vi "Main.vi"(8 "error in":errorcluster, 11 "UI Cam Basler in":refnum<class "UI Cam Basler.lvclass">) -> (0 "error out":errorcluster, 3 "UI Cam Basler out":refnum<class "UI Cam Basler.lvclass">)   [LabVIEW 2023, in "UI Cam Basler.lvclass"]
doc: "The Queued Message Handler of a Worker."
uses:
  UI Cam Basler.lvclass
  <vilib>/userDefined/High Color/IMAQdx.ctl
  C:/Program Files (x86)/National Instruments/LabVIEW 2023/vi.lib/addons/_Workers/Library/Classes/Worker/Worker.lvclass
  Data Image.ctl
  <vilib>/vision/Image Controls.llb/IMAQ Image.ctl
  UI Cam Basler.lvclass/UI Cam Basler.ctl
  <vilib>/addons/_Workers/Library/Classes/Worker/Worker.lvclass/Worker.ctl
  Initialization Data.ctl
  <vilib>/MGI/Panel Manager - .NET Panels/MDI/MDI Container/MDI Container.lvclass
  <vilib>/MGI/Panel Manager/Panel/Window Position/Reference Position/Alignment.ctl
  <vilib>/MGI/Panel Manager/Panel/Window Position/Reference Position/Horizontal Alignment.ctl
  <vilib>/MGI/Panel Manager/Panel/Window Position/Reference Position/Vertical Alignment.ctl
  <vilib>/MGI/Panel Manager/Panel/Window Position/Reference Position/Size/Reference Size/Reference Size.lvclass/Reference Size.ctl
  <vilib>/Utility/miscctls.llb/LVMinMaxIncTypeDef.ctl
  <vilib>/MGI/Panel Manager/Panel/Window Position/Reference Position/Size/Reference Size/Reference Size.vi
  <vilib>/MGI/Panel Manager/Panel/Window Position/Reference Position/Size/Reference Size/Reference Size.lvclass
  C:/Program Files (x86)/National Instruments/LabVIEW 2023/vi.lib/MGI/Panel Manager/Panel/Window Position/Reference Position/Size/Size.lvclass
  <vilib>/MGI/Panel Manager - .NET Panels/MDI/MDI Panel/MDI Panel.lvclass
  C:/Program Files (x86)/National Instruments/LabVIEW 2023/vi.lib/MGI/Panel Manager/Panel/Panel/Panel.lvclass
  Acq Cam Basler/Acq Cam Basler.lvclass
  <vilib>/MGI/Panel Manager - .NET Panels/MDI/MDI Panel/MDI Panel_Sized Window.vi
  <userlib>/LV-TOML/lib/Write TOML File (TOML).vi
  <vilib>/addons/_Workers/Library/Classes/Message/Enqueue Message to Queue.vi
  <vilib>/addons/_Workers/Library/Classes/Message/Enqueue Message to Self v2.vi
  <vilib>/addons/_Workers/Library/Classes/Worker/Worker.lvclass
  <vilib>/MGI/Panel Manager/Panel/Window Position/Reference Position/Reference Position.lvclass
  <vilib>/MGI/Panel Manager/Panel/Panel.lvlib
  <vilib>/MGI/Panel Manager/Panel/Panel/Panel.lvclass
  <userlib>/LV-TOML/lib/LV-TOML.lvlib
  <vilib>/addons/_Workers/Library/Classes/Message/Message.lvclass
  C:/Program Files (x86)/National Instruments/LabVIEW 2023/vi.lib/addons/_Workers/Library/Classes/Workers Object/Workers Object.lvclass
  C:/Users/flepetit/Desktop/CamView-mdi-LV/Workers/Acq Cam Basler/Acq Cam Basler.lvclass
  C:/Users/flepetit/Desktop/CamView-mdi-LV/Workers/UI Cam Basler/UI Cam Basler.lvclass
  C:/Program Files (x86)/National Instruments/LabVIEW 2023/vi.lib/MGI/Panel Manager/Panel/Panel/Window/Window.lvclass
  C:/Program Files (x86)/National Instruments/LabVIEW 2023/vi.lib/MGI/Panel Manager - .NET Panels/MDI/MDI Panel/MDI Panel.lvclass
  C:/Program Files (x86)/National Instruments/LabVIEW 2023/vi.lib/MGI/Panel Manager/Panel/Window Position/Reference Position/Size/Reference Size/Reference Size.lvclass
panel:
  out "Image":T1(plugin-control)
  in  "Commande onglets":T2(tab)
  in  "Save Config":bool
  in  "Start":bool
  in  "Stop":bool
  in  "Camera Name":T3
  out "FPS":dbl
  in  "Gain":dbl=100.0 min=100.0 max=1023.0 step=1.0
  in  "Shutter(us)":dbl=4.0 min=4.0 max=1000000.0 step=1.0
  in  "ROI":bool
  in  "toolbar?":bool
  in  "Palette":u32(ring)=5 items=["Grayscale", "Binary", "Gradient", "Rainbow", "Temperature", "User Defined", "Binary 16 Bit", "Gradient 16 Bit", "Rainbow 16 Bit", "Temperature 16 Bit", "User Defined 16 Bit"]
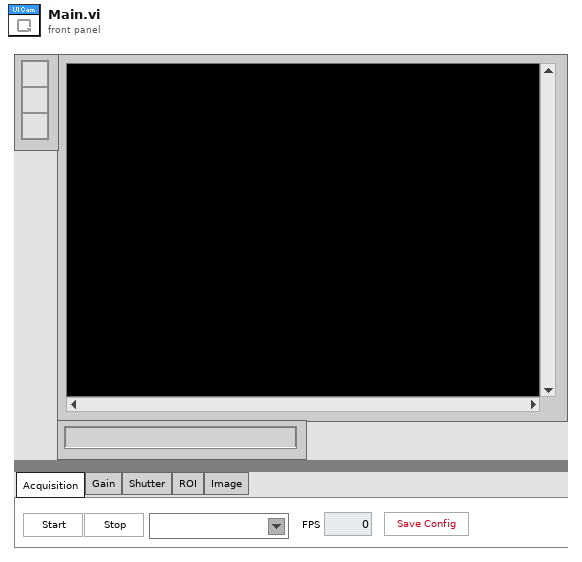
[diagram p1: front panel]
types:
  T1 = typedef "IMAQ Image.ctl" = refnum<image>
  T2 = enum32{"Acquisition", "Gain", "Shutter", "ROI", "Image"}
  T3 = typedef "IMAQdx.ctl" = refnum<k21>
  T4 = typedef "UI Cam Basler.lvclass/Data Image.ctl" = cluster{"Image Out":T1, "FPS":dbl}
  T5 = typedef "UI Cam Basler.lvclass/Initialization Data.ctl" = cluster{"Module Name":string, "Container":refnum<class "MDI Container.lvclass">, "Offset":cluster{"Horizontal":i16, "Vertical":i16}, "Width Scale":dbl, "Height Scale":dbl, "Alignment":T6}
  T6 = typedef "Panel.lvlib/Reference Position.lvclass/Alignment.ctl" = cluster{"Horizontal":T7, "Vertical":T8}
  T7 = typedef "Panel.lvlib/Reference Position.lvclass/Horizontal Alignment.ctl" = enum16{"Left", "Center", "Right"}
  T8 = typedef "Panel.lvlib/Reference Position.lvclass/Vertical Alignment.ctl" = enum16{"Top", "Center", "Bottom"}
  T9 = typedef "LVMinMaxIncTypeDef.ctl" = cluster{"Minimum":dbl, "Maximum":dbl, "Increment":dbl}
  T10 = typedef "UI Cam Basler.lvclass/Parsed Data Acquisition.ctl" = cluster{"Config Acquisition":cluster{"Camera name":string, "Gain":dbl, "Shutter(us)":dbl, "ROI":bool, "ROI coor":T11, "Palette":u32, "ModelName":string}}
  T11 = typedef "IMAQ Rectangle" = cluster{"Left":i32, "Top":i32, "Right":i32, "Bottom":i32, "Rotation":dbl}
  T12 = typedef "LV-TOML.lvlib/TOML Value.ctl" = cluster{"type":enum16{"Table", "Array", "String", "Integer", "Float", "Boolean", "Offset Date-Time", "Local Date-Time", "Local Date", "Local Time", "Path"}, "value":variant}
  T13 = typedef "Workers.lvlib/Case Label.ctl" = string
  T14 = typedef "ROI Descriptor" = cluster{"Global Rectangle":i32[], "Contours":cluster{"ID":enum32{"External", "Internal"}, "Type":u32, "Coordinates":i32[]}[]}
  T15 = cluster{"Global Rectangle":i32[], "Contours":cluster{"Contour Type":u32, "ROI Type":u32, "Points":i32[]}[]}
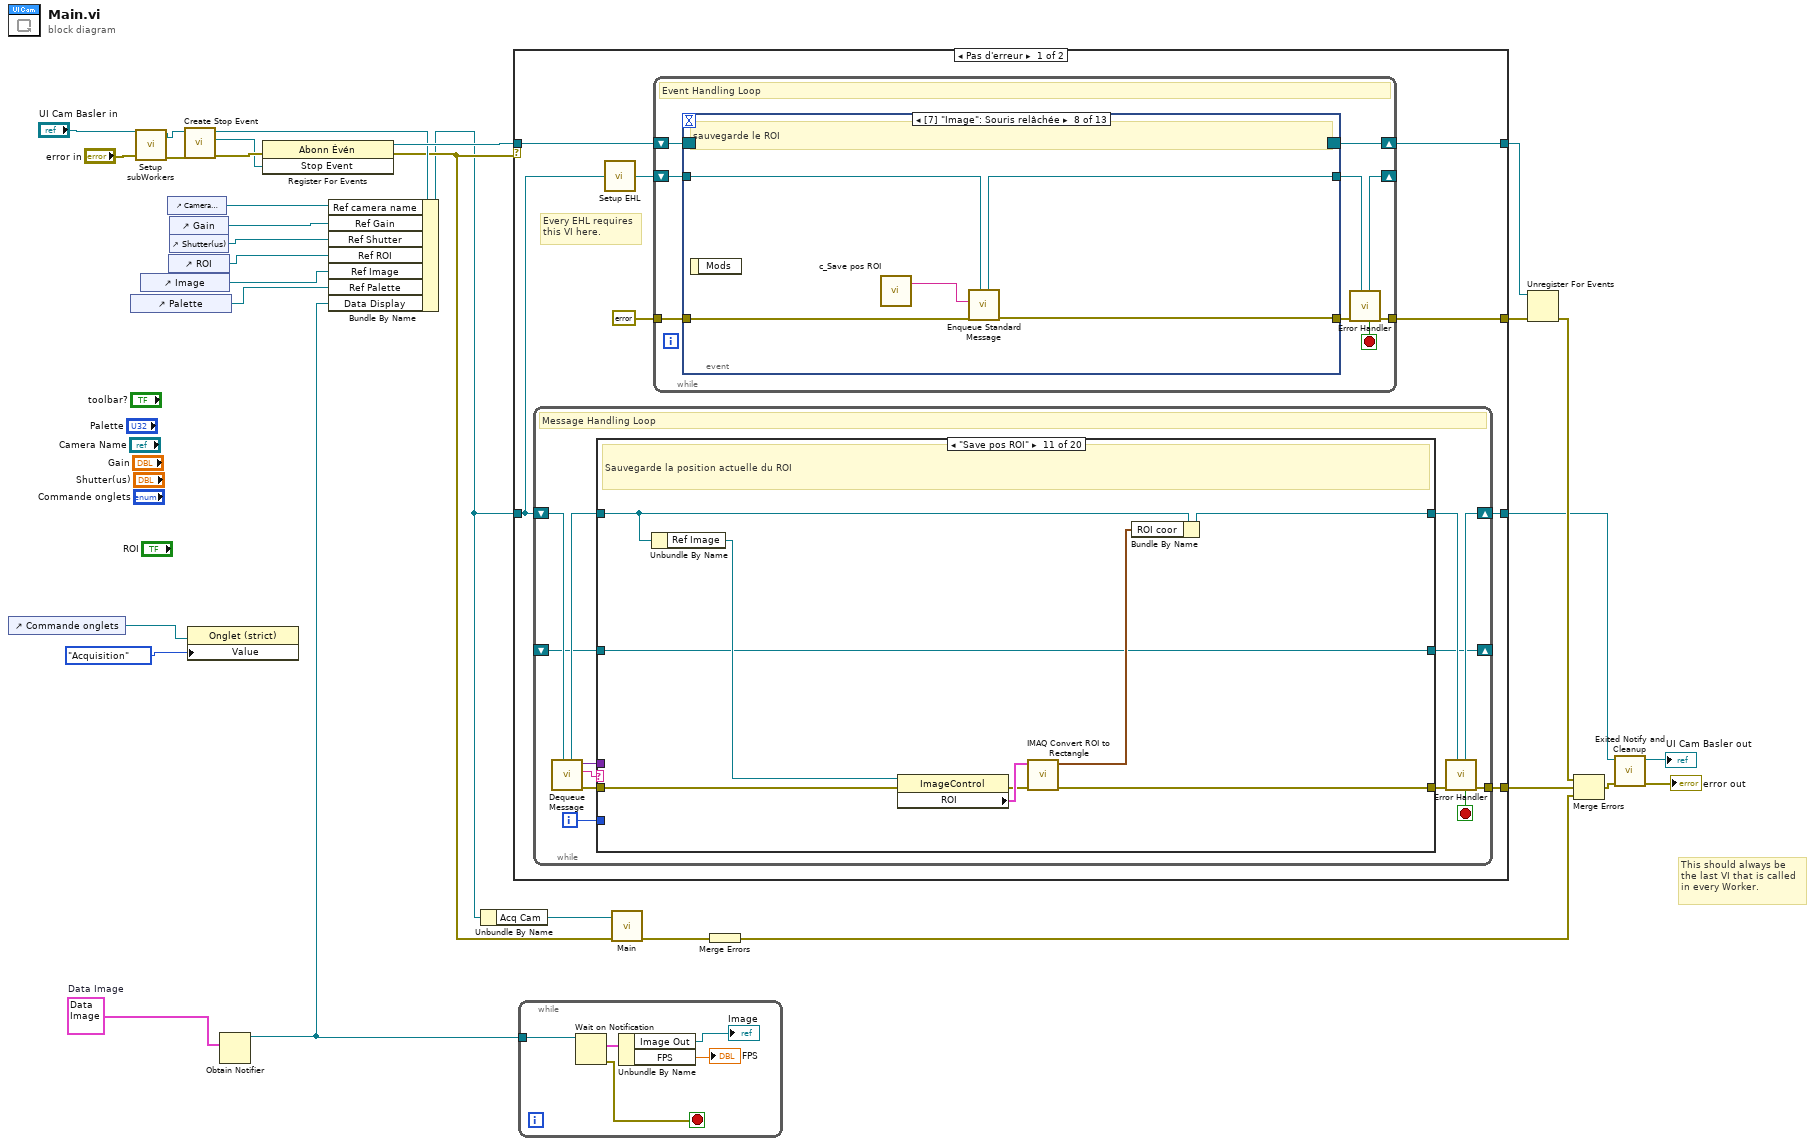
[diagram p0: block diagram]
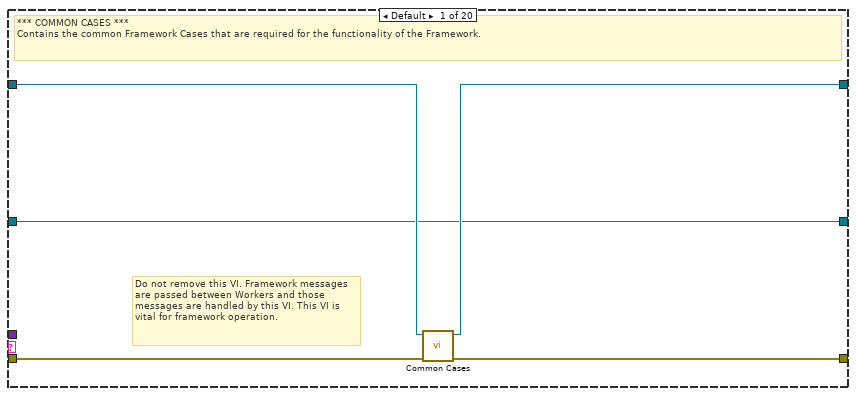
[diagram p2: hidden frame]
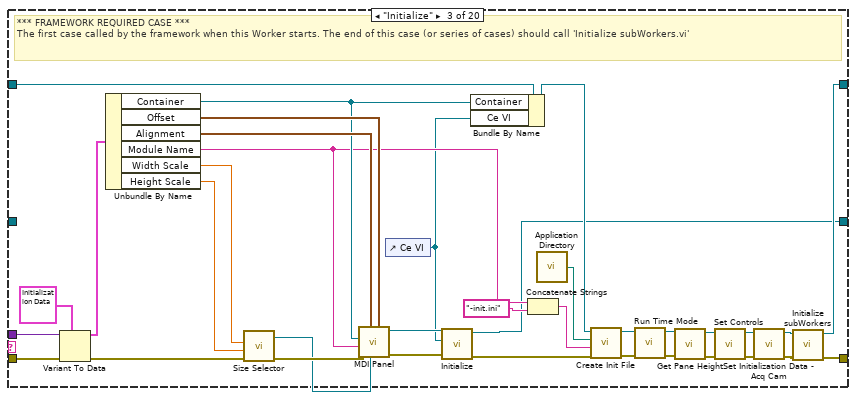
[diagram p4: hidden frame]
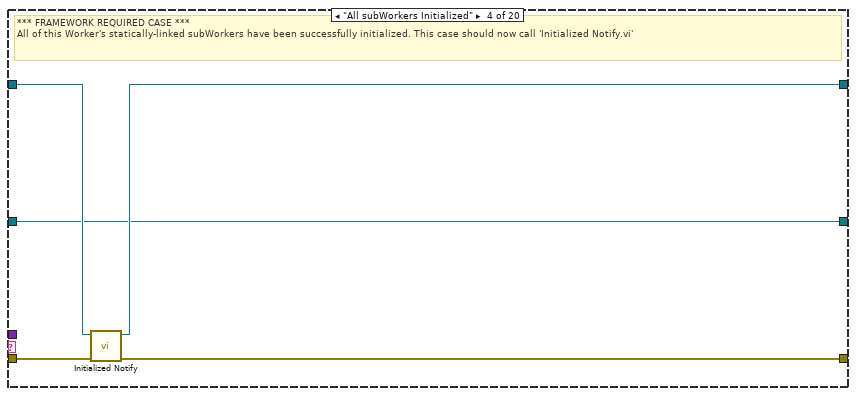
[diagram p5: hidden frame]
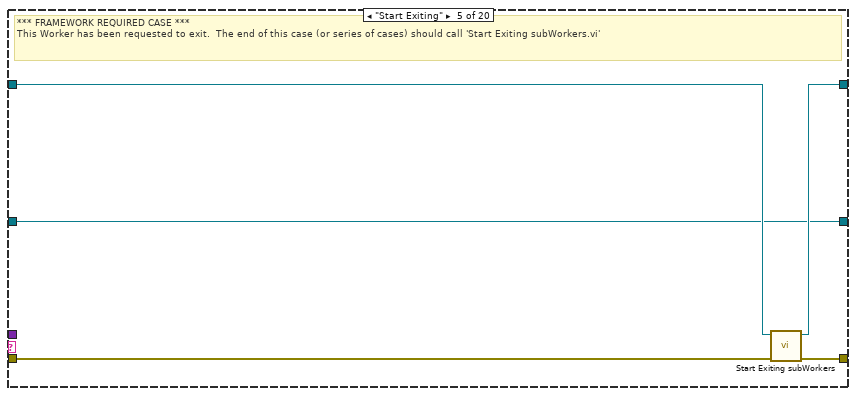
[diagram p6: hidden frame]
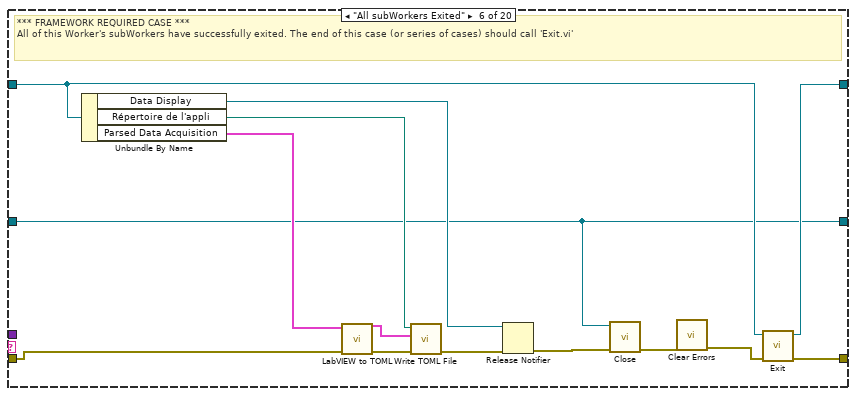
[diagram p7: hidden frame]
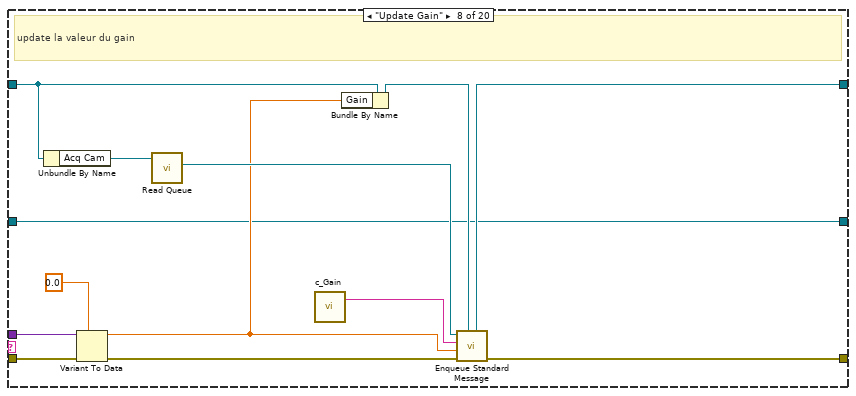
[diagram p9: hidden frame]
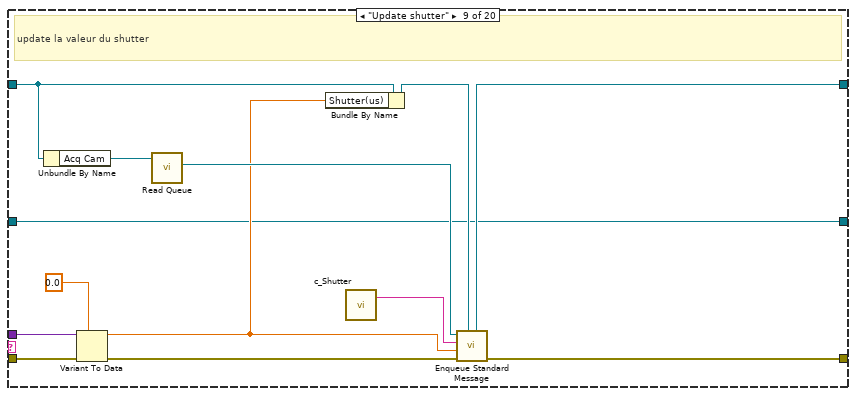
[diagram p10: hidden frame]
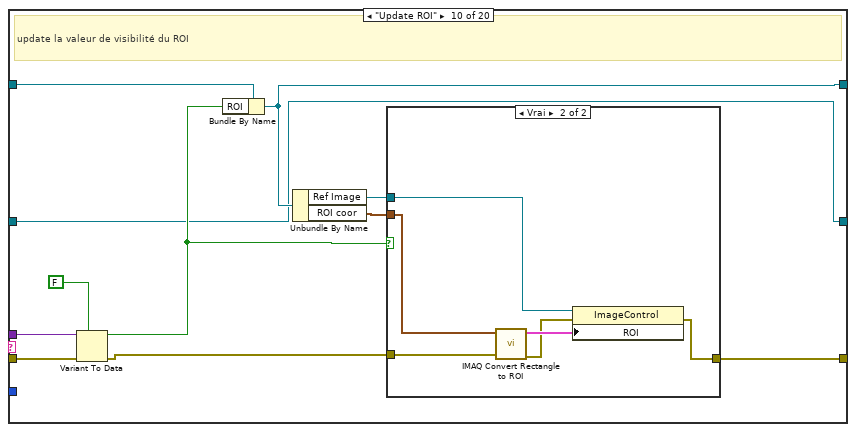
[diagram p11: hidden frame]
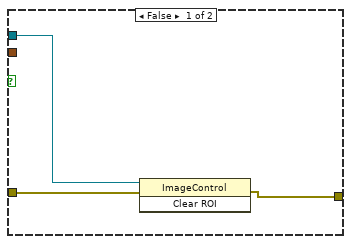
[diagram p12: hidden frame]
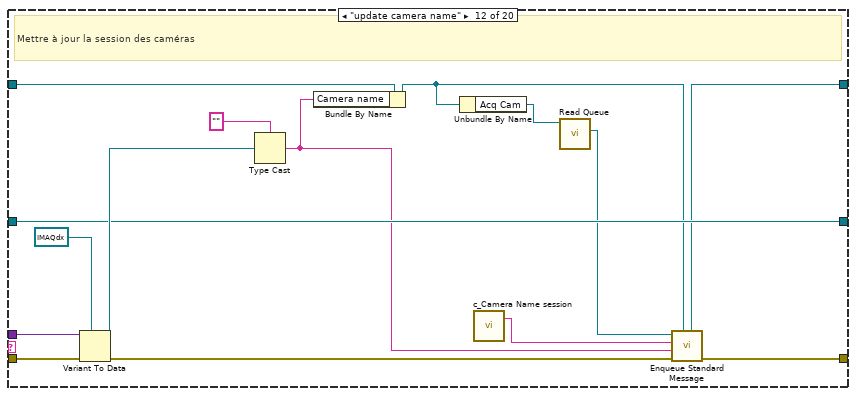
[diagram p13: hidden frame]
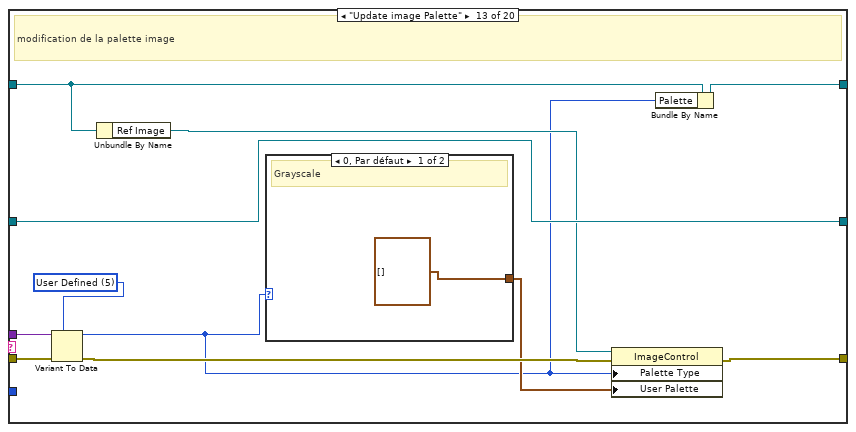
[diagram p14: hidden frame]
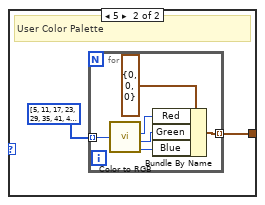
[diagram p15: hidden frame]
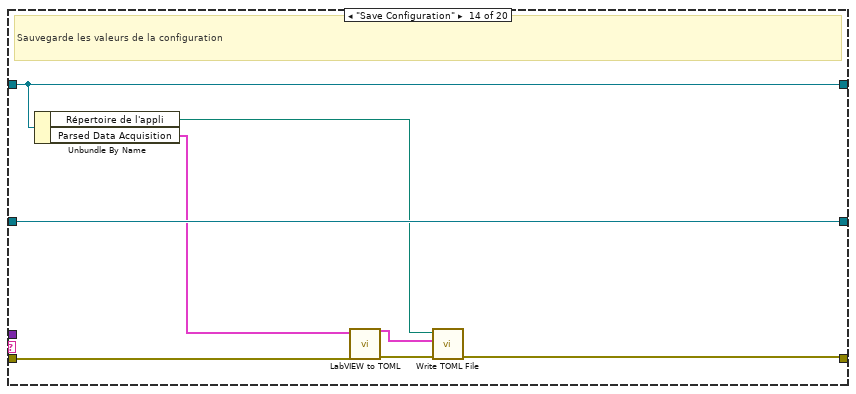
[diagram p16: hidden frame]
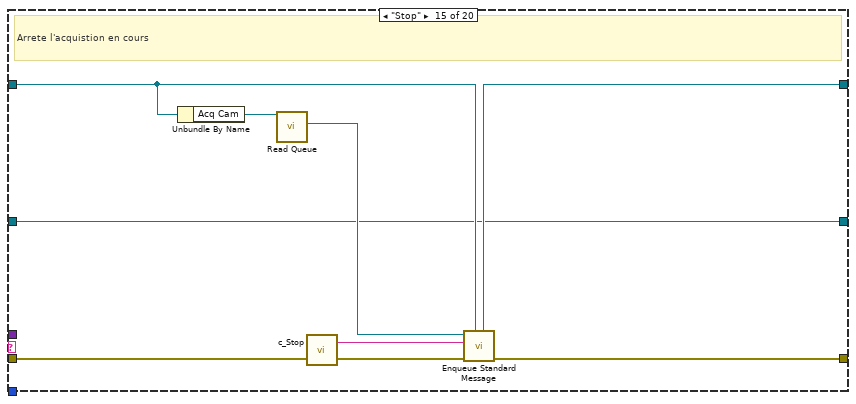
[diagram p17: hidden frame]
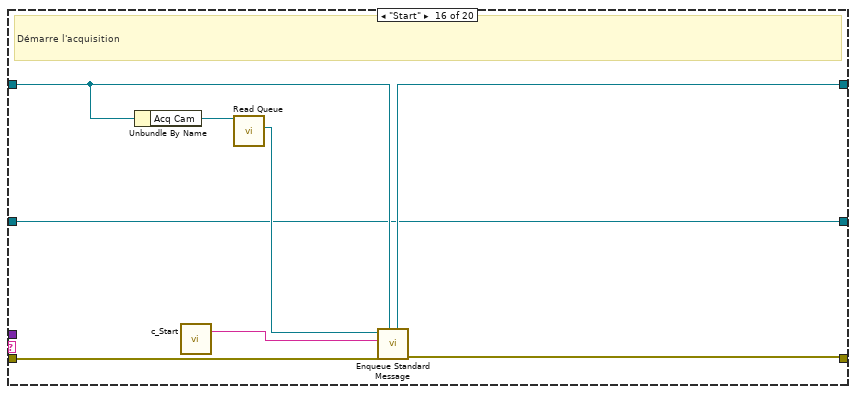
[diagram p18: hidden frame]
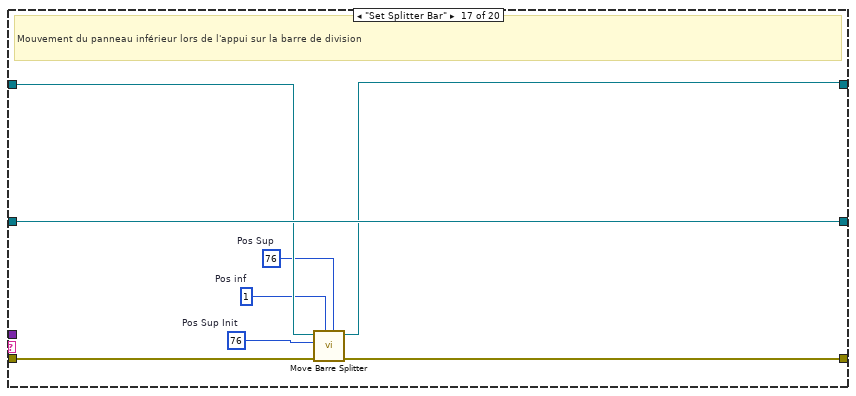
[diagram p19: hidden frame]
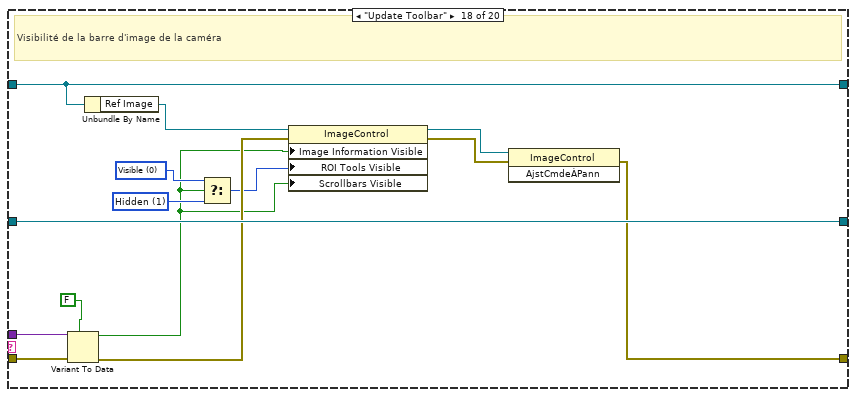
[diagram p20: hidden frame]
diagram:
  w13 = T4 {"Image Out"=refnum, "FPS"=0.0}  # Data Image
  # "This should always be the last VI that is called in every Worker."
  n1 = control-ref of="Commande onglets"() -> (w6:refnum<vi>)
  n2 = control-ref of="Palette"() -> (w7:refnum<vi>)
  n3 = call "Setup subWorkers.vi"("error in"="error in", "UI Cam Basler in"="UI Cam Basler in") -> ("error out"=w20:errorcluster, "UI Cam Basler out"=w21:refnum<class "UI Cam Basler.lvclass">)  [unwired: 8 in]
  n4 = control-ref of="Image"() -> (w8:refnum<vi>)
  n5 = control-ref of="Camera Name"() -> (w14:refnum<vi>)
  n6 = control-ref of="ROI"() -> (w9:refnum<vi>)
  n7 = control-ref of="Gain"() -> (w11:refnum<vi>)
  n8 = control-ref of="Shutter(us)"() -> (w10:refnum<vi>)
  n9 = call-dynamic "Create Stop Event.vi"("error in"=w20, "Worker"=w21) -> ("error out"=w26:errorcluster, "Stop Event"=w23:refnum<user-event>, "Worker out"=w17:refnum<class "UI Cam Basler.lvclass">)  [unwired: 7 in]
  n10 = property class="Onglet (strict)"(reference=w6, "Value"=T2."Acquisition" ("Commande onglets")) -> ()  [unwired: 1 in, 2 out]
  n11 = Obtain Notifier(notification data type=w13) -> (notifier out=w12:refnum<notifier>)  [unwired: 3 in, 2 out]
  n12 = register-events(error in=w26, w23) -> (reference out=w25:refnum<event-registration>, error out=w16:errorcluster)  [unwired: 1 in]
  n13 = Bundle By Name(cluster=w17, "Ref camera name"=w14, "Ref Gain"=w11, "Ref Shutter"=w10, "Ref ROI"=w9, "Ref Image"=w8, "Ref Palette"=w7, "Data Display"=w12) -> (w15:refnum<class "UI Cam Basler.lvclass">)
  n14 = Unbundle By Name(w15) -> ("Acq Cam"=w22:refnum<class "Acq Cam Basler.lvclass">)
  n15 = case shown="Pas d'erreur" w16 {
    tunnel: w15 -> [w34 w413]
    tunnel: [w32 w414] -> w24
    tunnel: w25 -> [w39 w415]
    tunnel: [w36 w416] -> w30
    tunnel: [w38 w415] -> w29
    tunnel: [w33 w412] -> w27
    selector: w16 -> [_ w416]
    frame No Error {
      # "Every EHL requires\nthis VI here."
      n16 = while {
        shift-right: [w50] -> w33
        shift-left: w34 -> [w52]
        tunnel: [w51] -> w32
        shift-right: [w41] -> _
        shift-left: _ -> [w40]
        i -> [w42]
        stop <- w43 stop-if-true
        # "Message Handling Loop"
        n17 = call-dynamic "Dequeue Message.vi"("Worker"=w52) -> ("error out"=w49:errorcluster, "Case out"=w44:string, "Data out"=w45:variant, "Worker out"=w47:refnum<class "UI Cam Basler.lvclass">)  [unwired: 6 in, 1 out]
        n18 = case "Worker MHL Case Structure (DO NOT CHANGE LABEL NAME)" shown="\"Save pos ROI\"" w44 {
          tunnel: w49 -> [w57 w59 w93 w98 w102 w110 w121 w135 w148 w159 w175 w191 w202 w217 w226 w236 w243 w255 w260 w269]
          tunnel: [w56 w59 w95 w97 w105 w119 w121 w130 w144 w151 w174 w184 w197 w216 w225 w235 w242 w246 w260 w262] -> w48
          tunnel: w47 -> [w55 w60 w92 w100 w103 w117 w122 w128 w142 w156 w173 w192 w199 w215 w223 w233 w241 w257 w261 w271]
          tunnel: [w54 w60 w94 w99 w104 w118 w122 w129 w143 w154 w171 w179 w194 w215 w224 w234 w240 w257 w261 w265] -> w46
          tunnel: w45 -> [_ _ w91 _ _ _ _ w134 w147 w158 _ w190 w201 _ _ _ _ w254 _ w268]
          tunnel: w42 -> [_ _ _ _ _ _ _ _ _ _ _ _ _ _ _ _ _ _ _ _]
          tunnel: [w53 w58 w68 w96 w101 w108 w120 w123 w136 w149 w169 w186 w203 w220 w221 w229 w244 w258 w259 w270] -> w41
          tunnel: w40 -> [w53 w58 _ w96 w101 w108 w120 w123 w136 w149 w169 w186 w203 w220 w221 w229 w244 w258 w259 w270]
          frame Default {
            # "Do not remove this VI. Framework messages are passed between Workers and those messages are handled by this VI. This VI is vital for framework operation."
            # "*** COMMON CASES ***\nContains the common Framework Cases that are required for the functionality of the Framework."
            n19 = call-dynamic "Common Cases.vi"("error in"=w57, "Worker in"=w55) -> ("error out"=w56:errorcluster, "Worker out"=w54:refnum<class "UI Cam Basler.lvclass">)  [unwired: 8 in]
          }
          frame "------ FRAMEWORK REQUIRED CASES ------" {
            # "Start of Framework Required Cases"
          }
          frame "Initialize" {
            # "*** FRAMEWORK REQUIRED CASE ***\nThe first case called by the framework when this Worker starts. The end of this case (or series of cases) should call 'Initialize subWorkers.vi'"
            n20 = Variant To Data(error in=w93, type=T5 {"Module Name"="", "Container"=refnum, "Offset"={"Horizontal"=0, "Vertical"=0}, "Width Scale"=300.0, "Height Scale"=500.0, "Alignment"={"Horizontal"=enum."Left", "Vertical"=enum."Top"}} ("Initialization Data"), Variant=w91) -> (data=w89:T5, error out=w88:errorcluster)
            n21 = Unbundle By Name(w89) -> ("Container"=w79:refnum<class "MDI Container.lvclass">, "Offset"=w81:cluster{"Horizontal":i16, "Vertical":i16}, "Alignment"=w82:T6, "Module Name"=w75:string, "Width Scale"=w85:dbl, "Height Scale"=w84:dbl)
            n22 = call-poly <vilib>:"Size Selector.vi"("Error In"=w88, "Height Scale"=w84, "Width Scale"=w85) -> ("Error Out"=w87:errorcluster, "Static Out"=w83:refnum<class "Reference Size.lvclass">)  [unwired: 7 in]
            n23 = call-poly <vilib>:"MDI Panel.vi"("Offset"=w81, "Size"=w83, "Alignment"=w82, "error in (no error)"=w87, "Title"=w75, "MDI Container"=w79) -> ("error out"=w86:errorcluster, "MDI Panel out"=w80:refnum<class "MDI Panel.lvclass">)  [unwired: 4 in]
            n24 = control-ref of="Ce VI"() -> (w65:refnum<vi>)
            n25 = call <vilib>:"Initialize.vi"("error in (no error)"=w86, "VI Refnum"=w65, "Panel In"=w80) -> ("error out"=w78:errorcluster, "Panel Out"=w68:refnum<class "MDI Panel.lvclass">)  [unwired: 6 in, 1 out]
            n26 = Bundle By Name(cluster=w92, "Container"=w79, "Ce VI"=w65) -> (w73:refnum<class "UI Cam Basler.lvclass">)
            n27 = Concatenate Strings(w75, "-init.ini") -> (w74:string)
            n28 = call <vilib>:"Application Directory.vi"() -> ("Application Directory"=w76:path)
            n29 = call "Create Init File.vi"("error in (no error)"=w78, "Nom du fichier ini"=w74, "Répertoire de l'appli"=w76, "UI Cam Basler in"=w73) -> ("error out"=w66:errorcluster, "UI Cam Basler out"=w67:refnum<class "UI Cam Basler.lvclass">)  [unwired: 6 in]
            n30 = call "Run Time Mode.vi"("error in (no error)"=w66, "UI Cam Basler en entrée"=w67) -> ("error out"=w62:errorcluster, "UI Cam Basler en sortie"=w64:refnum<class "UI Cam Basler.lvclass">)  [unwired: 8 in]
            n31 = call "Get Pane Height.vi"("error in (no error)"=w62, "UI Cam Basler en entrée"=w64) -> ("error out"=w61:errorcluster, "UI Cam Basler en sortie"=w63:refnum<class "UI Cam Basler.lvclass">)  [unwired: 8 in]
            n32 = call "Set Controls.vi"("error in (no error)"=w61, "UI Cam Basler en entrée"=w63) -> ("error out"=w69:errorcluster, "UI Cam Basler en sortie"=w70:refnum<class "UI Cam Basler.lvclass">)  [unwired: 8 in]
            n33 = call "Set Initialization Data - Acq Cam.vi"("error in"=w69, "UI Cam Basler in"=w70) -> ("error out"=w72:errorcluster, "UI Cam Basler out"=w71:refnum<class "UI Cam Basler.lvclass">)  [unwired: 8 in]
            n34 = call-dynamic "Initialize subWorkers.vi"("error in"=w72, "Worker"=w71) -> ("error out"=w95:errorcluster, "dup Worker out"=w94:refnum<class "UI Cam Basler.lvclass">)  [unwired: 8 in]
          }
          frame "All subWorkers Initialized" {
            # "*** FRAMEWORK REQUIRED CASE ***\nAll of this Worker's statically-linked subWorkers have been successfully initialized. This case should now call 'Initialized Notify.vi'"
            n35 = call-dynamic "Initialized Notify.vi"("error in"=w98, "Worker"=w100) -> ("error out"=w97:errorcluster, "dup Worker out"=w99:refnum<class "UI Cam Basler.lvclass">)  [unwired: 8 in]
          }
          frame "Start Exiting" {
            # "*** FRAMEWORK REQUIRED CASE ***\nThis Worker has been requested to exit.  The end of this case (or series of cases) should call 'Start Exiting subWorkers.vi'"
            n36 = call-dynamic "Start Exiting subWorkers.vi"("error_in"=w102, "Worker"=w103) -> ("error out"=w105:errorcluster, "dup Worker out"=w104:refnum<class "UI Cam Basler.lvclass">)  [unwired: 8 in]
          }
          frame "All subWorkers Exited" {
            # "*** FRAMEWORK REQUIRED CASE ***\nAll of this Worker's subWorkers have successfully exited. The end of this case (or series of cases) should call 'Exit.vi'"
            n37 = Unbundle By Name(w117) -> ("Data Display"=w111:refnum<notifier>, "Répertoire de l'appli"=w113:path, "Parsed Data Acquisition"=w114:T10)
            n38 = call <userlib>:"LabVIEW to TOML.vi"("error in (no error)"=w110, "LV Value"=w114) -> ("error out"=w115:errorcluster, "TOML Value"=w116:T12)  [unwired: 7 in, 1 out]
            n39 = call-poly <userlib>:"Write TOML File.vi"("error in (no error)"=w115, "Value"=w116, "file path (use dialog)"=w113) -> ("error out"=w112:errorcluster)  [unwired: 8 in]
            n40 = Release Notifier(notifier=w111, error in (no error)=w112) -> (error out=w109:errorcluster)  [unwired: 1 in, 2 out]
            n41 = call-dynamic "Close.vi"("error in (no error)"=w109, "MDI Child in"=w108) -> ("error out"=w107:errorcluster)  [unwired: 9 in]
            n42 = call <vilib>:"Clear Errors.vi"("error in (no error)"=w107) -> ("error out"=w106:errorcluster)  [unwired: 5 in, 1 out]
            n43 = call-dynamic "Exit.vi"("error_in"=w106, "Worker"=w117) -> ("error out"=w119:errorcluster, "dup Worker out"=w118:refnum<class "UI Cam Basler.lvclass">)  [unwired: 8 in]
          }
          frame "--------Messages--Himself------------------------" {
            # "End of Framework Required Cases"
          }
          frame "Update Gain" {
            # "update la valeur du gain"
            n44 = Unbundle By Name(w128) -> ("Acq Cam"=w127:refnum<class "Acq Cam Basler.lvclass">)
            n45 = Variant To Data(error in=w135, type=0.0, Variant=w134) -> (data=w124:dbl, error out=w131:errorcluster)
            n46 = call <vilib>:"Read Queue.vi"("Worker"=w127) -> ("Message Queue out"=w126:refnum<class "Message Queue.lvclass">)  [unwired: 9 in, 1 out]
            n47 = call "c_Gain.vi"() -> ("Case Label"=w132:T13)  [unwired: 1 in]
            n48 = Bundle By Name(cluster=w128, "Gain"=w124) -> (w125:refnum<class "UI Cam Basler.lvclass">)
            n49 = call-poly <vilib>:"Enqueue Standard Message.vi"("Worker"=w125, "error in"=w131, "Data"=w124, "Case Label"=w132, "Message Queue"=w126) -> ("error out"=w130:errorcluster, "dup Worker out"=w129:refnum<class "UI Cam Basler.lvclass">)  [unwired: 4 in, 1 out]
          }
          frame "Update shutter" {
            # "update la valeur du shutter"
            n50 = Unbundle By Name(w142) -> ("Acq Cam"=w141:refnum<class "Acq Cam Basler.lvclass">)
            n51 = Variant To Data(error in=w148, type=0.0, Variant=w147) -> (data=w138:dbl, error out=w145:errorcluster)
            n52 = call <vilib>:"Read Queue.vi"("Worker"=w141) -> ("Message Queue out"=w140:refnum<class "Message Queue.lvclass">)  [unwired: 9 in, 1 out]
            n53 = Bundle By Name(cluster=w142, "Shutter(us)"=w138) -> (w139:refnum<class "UI Cam Basler.lvclass">)
            n54 = call "c_Shutter.vi"() -> ("Case Label"=w137:T13)  [unwired: 1 in]
            n55 = call-poly <vilib>:"Enqueue Standard Message.vi"("Worker"=w139, "error in"=w145, "Data"=w138, "Case Label"=w137, "Message Queue"=w140) -> ("error out"=w144:errorcluster, "dup Worker out"=w143:refnum<class "UI Cam Basler.lvclass">)  [unwired: 4 in, 1 out]
          }
          frame "Update ROI" {
            # "update la valeur de visibilité du ROI"
            n56 = Variant To Data(error in=w159, type=FALSE, Variant=w158) -> (data=w155:bool, error out=w152:errorcluster)
            n57 = Bundle By Name(cluster=w156, "ROI"=w155) -> (w154:refnum<class "UI Cam Basler.lvclass">)
            n58 = Unbundle By Name(w154) -> ("Ref Image"=w150:refnum<vi>, "ROI coor"=w153:T11)
            n59 = case shown="Vrai" w155 {
              tunnel: w153 -> [_ w168]
              tunnel: w152 -> [w162 w167]
              tunnel: [w161 w163] -> w151
              tunnel: w150 -> [w160 w166]
              frame False {
                n60 = invoke class="ImageControl" method="Clear ROI"(reference=w160, error in=w162) -> (error out=w161:errorcluster)  [unwired: 1 in, 2 out]
              }
              frame True {
                n61 = call "IMAQ Convert Rectangle to ROI"("error in (no error)"=w167, "Rectangle"=w168) -> ("error out"=w164:errorcluster, "ROI Descriptor"=w165:T14)  [unwired: 7 in]
                n62 = property class="ImageControl"(reference=w166, error in=w164, "ROI"=w165) -> (error out=w163:errorcluster)  [unwired: 1 out]
              }
            }
          }
          frame "Save pos ROI" {
            # "Sauvegarde la position actuelle du ROI"
            n63 = Unbundle By Name(w173) -> ("Ref Image"=w172:refnum<vi>)
            n64 = property class="ImageControl"(reference=w172, error in=w175) -> (error out=w176:errorcluster, "ROI"=w177:T15)  [unwired: 1 out]
            n65 = call "IMAQ Convert ROI to Rectangle"("error in (no error)"=w176, "ROI Descriptor"=w177) -> ("error out"=w174:errorcluster, "Rectangle"=w170:T11)  [unwired: 7 in]
            n66 = Bundle By Name(cluster=w173, "ROI coor"=w170) -> (w171:refnum<class "UI Cam Basler.lvclass">)
          }
          frame "update camera name" {
            # "Mettre à jour la session des caméras"
            n67 = Variant To Data(error in=w191, type=T3 refnum ("Camera Name 2"), Variant=w190) -> (data=w188:T3, error out=w185:errorcluster)
            n68 = Type Cast(type="", x=w188) -> (*(type *) &x=w183:string)
            n69 = Bundle By Name(cluster=w192, "Camera name"=w183) -> (w180:refnum<class "UI Cam Basler.lvclass">)
            n70 = Unbundle By Name(w180) -> ("Acq Cam"=w182:refnum<class "Acq Cam Basler.lvclass">)
            n71 = call "c_Camera Name session.vi"() -> ("Case Label"=w178:T13)  [unwired: 1 in]
            n72 = call <vilib>:"Read Queue.vi"("Worker"=w182) -> ("Message Queue out"=w181:refnum<class "Message Queue.lvclass">)  [unwired: 9 in, 1 out]
            n73 = call-poly <vilib>:"Enqueue Standard Message.vi"("Worker"=w180, "error in"=w185, "Data"=w183, "Case Label"=w178, "Message Queue"=w181) -> ("error out"=w184:errorcluster, "dup Worker out"=w179:refnum<class "UI Cam Basler.lvclass">)  [unwired: 4 in, 1 out]
          }
          frame "Update image Palette" {
            w200 = u32 5 items=["Grayscale", "Binary", "Gradient", "Rainbow", "Temperature", "User Defined", "Binary 16 Bit", "Gradient 16 Bit", "Rainbow 16 Bit", "Temperature 16 Bit", "User Defined 16 Bit"] ("Palette 2")
            # "modification de la palette image"
            n74 = Variant To Data(error in=w202, type=w200, Variant=w201) -> (data=w193:u32, error out=w198:errorcluster)
            n75 = Unbundle By Name(w199) -> ("Ref Image"=w196:refnum<vi>)
            n76 = case shown="0, Par défaut" w193 {
              tunnel: [cluster{"Red":u8, "Green":u8, "Blue":u8}[] [] w206] -> w195
              frame 0, Default {
                # "Grayscale"
              }
              frame 5 {
                # "User Color Palette"
                n77 = for {
                  tunnel: u32[] [5, 11, 17, 23, 29, 35, 41, 47, 53, 59, 65, 71, 77, 83, 89, 95, 101, 107, 113, 119, 125, 131, 137, 143, 149, 155, 161, 167, 173, 179, 185, 191, 197, 203, 209, 215, 221, 227, 233, 239, 245, 251, 511, 2047, 3583, 5119, 6655, 8191, 9727, 11263, 12799, 14335, 15871, 17407, 18943, 20479, 22015, 23551, 25087, 26623, 28159, 29695, 31231, 32767, 34303, 35839, 37375, 38911, 40447, 41983, 43519, 45055, 46591, 48127, 49663, 51199, 52735, 54271, 55807, 57343, 58879, 60415, 61951, 63487, 65023, 65532, 65526, 65520, 65514, 65508, 65502, 65496, 65490, 65484, 65478, 65472, 65466, 65460, 65454, 65448, 65442, 65436, 65430, 65424, 65418, 65412, 65406, 65400, 65394, 65388, 65382, 65376, 65370, 65364, 65358, 65352, 65346, 65340, 65334, 65328, 65322, 65316, 65310, 65304, 65298, 65292, 65286, 65280, 130816, 130816, 130816, 130816, 130816, 130816, 130816, 130816, 130816, 130816, 130816, 130816, 130816, 130816, 130816, 130816, 130816, 130816, 130816, 130816, 130816, 130816, 130816, 130816, 130816, 130816, 130816, 130816, 130816, 130816, 130816, 130816, 130816, 130816, 130816, 130816, 130816, 130816, 130816, 130816, 130816, 130816, 16776704, 16775168, 16773632, 16772096, 16770560, 16769024, 16767488, 16765952, 16764416, 16762880, 16761344, 16759808, 16758272, 16756736, 16755200, 16753664, 16752128, 16750592, 16749056, 16747520, 16745984, 16744448, 16742912, 16741376, 16739840, 16738304, 16736768, 16735232, 16733696, 16732160, 16730624, 16729088, 16727552, 16726016, 16724480, 16722944, 16721408, 16719872, 16718336, 16716800, 16715264, 16713728, 16712192, 16712451, 16713993, 16715535, 16717077, 16718619, 16720161, 16721703, 16723245, 16724787, 16726329, 16727871, 16729413, 16730955, 16732497, 16734039, 16735581, 16737123, 16738665, 16740207, 16741749, 16743291, 16744833, 16746375, 16747917, 16749459, 16751001, 16752543, 16754085, 16755627, 16757169, 16758711, 16760253, 16761795, 16763337, 16764879, 16766421, 16767963, 16769505, 16771047, 16772589, 16774131, 16775673, 16777215] ("tableau ajouté 3") -> [w208] mode=indexing
                  tunnel: [w207] -> w206 mode=indexing
                  n78 = call <vilib>:"Color to RGB.vi"("Color"=w208) -> ("R"=w211:u8, "G"=w210:u8, "B"=w209:u8)  [unwired: 1 out]
                  n79 = Bundle By Name(cluster=cluster{"Red":u8, "Green":u8, "Blue":u8} {"Red"=0, "Green"=0, "Blue"=0}, "Red"=w211, "Green"=w210, "Blue"=w209) -> (w207:cluster{"Red":u8, "Green":u8, "Blue":u8})
                }
              }
            }
            n80 = property on="Nœud de propriété" class="ImageControl"(reference=w196, error in=w198, "Palette Type"=w193, "User Palette"=w195) -> (error out=w197:errorcluster)  [unwired: 1 out]
            n81 = Bundle By Name(cluster=w199, "Palette"=w193) -> (w194:refnum<class "UI Cam Basler.lvclass">)
          }
          frame "Save Configuration" {
            # "Sauvegarde les valeurs de la configuration"
            n82 = Unbundle By Name(w215) -> ("Répertoire de l'appli"=w213:path, "Parsed Data Acquisition"=w214:T10)
            n83 = call <userlib>:"LabVIEW to TOML.vi"("error in (no error)"=w217, "LV Value"=w214) -> ("error out"=w218:errorcluster, "TOML Value"=w219:T12)  [unwired: 7 in, 1 out]
            n84 = call-poly <userlib>:"Write TOML File.vi"("error in (no error)"=w218, "Value"=w219, "file path (use dialog)"=w213) -> ("error out"=w216:errorcluster)  [unwired: 8 in]
          }
          frame "Stop" {
            # "Arrete l'acquistion en cours"
            n85 = Unbundle By Name(w223) -> ("Acq Cam"=w228:refnum<class "Acq Cam Basler.lvclass">)
            n86 = call <vilib>:"Read Queue.vi"("Worker"=w228) -> ("Message Queue out"=w227:refnum<class "Message Queue.lvclass">)  [unwired: 9 in, 1 out]
            n87 = call "c_Stop.vi"() -> ("Case Label"=w222:T13)  [unwired: 1 in]
            n88 = call-poly <vilib>:"Enqueue Standard Message.vi"("Worker"=w223, "error in"=w226, "Case Label"=w222, "Message Queue"=w227) -> ("error out"=w225:errorcluster, "dup Worker out"=w224:refnum<class "UI Cam Basler.lvclass">)  [unwired: 5 in, 1 out]
          }
          frame "Start" {
            # "Démarre l'acquisition"
            n89 = Unbundle By Name(w233) -> ("Acq Cam"=w232:refnum<class "Acq Cam Basler.lvclass">)
            n90 = call "c_Start.vi"() -> ("Case Label"=w230:T13)  [unwired: 1 in]
            n91 = call <vilib>:"Read Queue.vi"("Worker"=w232) -> ("Message Queue out"=w231:refnum<class "Message Queue.lvclass">)  [unwired: 9 in, 1 out]
            n92 = call-poly <vilib>:"Enqueue Standard Message.vi"("Worker"=w233, "error in"=w236, "Case Label"=w230, "Message Queue"=w231) -> ("error out"=w235:errorcluster, "dup Worker out"=w234:refnum<class "UI Cam Basler.lvclass">)  [unwired: 5 in, 1 out]
          }
          frame "Set Splitter Bar" {
            w237 = u32 76  # Pos Sup Init
            w239 = u32 1  # Pos inf
            w238 = u32 76  # Pos Sup
            # "Mouvement du panneau inférieur lors de l'appui sur la barre de division"
            n93 = call "Move Barre Splitter.vi"("Pos Sup"=w238, "Pos inf"=w239, "error in (no error)"=w243, "Pos Sup Init"=w237, "UI Cam Basler en entrée"=w241) -> ("error out"=w242:errorcluster, "UI Cam Basler en sortie"=w240:refnum<class "UI Cam Basler.lvclass">)  [unwired: 5 in]
          }
          frame "Update Toolbar" {
            w250 = u32 1 items=["Visible", "Hidden", "Hidden, Use WindTools Palette"] ("ROI Tools Visible")
            w251 = u32 0 items=["Visible", "Hidden", "Hidden, Use WindTools Palette"] ("ROI Tools Visible")
            # "Visibilité de la barre d'image de la caméra"
            n94 = Variant To Data(error in=w255, type=FALSE, Variant=w254) -> (data=w245:bool, error out=w252:errorcluster)
            n95 = Unbundle By Name(w257) -> ("Ref Image"=w256:refnum<vi>)
            n96 = Select(t=w251, s=w245, f=w250) -> (s? t:f=w249:u32)
            n97 = property class="ImageControl"(reference=w256, error in=w252, "Image Information Visible"=w245, "ROI Tools Visible"=w249, "Scrollbars Visible"=w245) -> (reference out=w248:refnum<vi>, error out=w247:errorcluster)
            n98 = invoke class="ImageControl" method="AjstCmdeÀPann"(reference=w248, error in=w247) -> (error out=w246:errorcluster)  [unwired: 1 in, 2 out]
          }
          frame "--------From Acq Cam Basler-----------------" {
            # "End of Framework Required Cases"
          }
          frame "ModelName" {
            # "Nom du modèle de la caméra"
            n99 = Variant To Data(error in=w269, type="", Variant=w268) -> (data=w266:string, error out=w263:errorcluster)
            n100 = Bundle By Name(cluster=w271, "ModelName"=w266) -> (w265:refnum<class "UI Cam Basler.lvclass">)
            n101 = Unbundle By Name(w265) -> ("Ref Gain"=w264:refnum<vi>)
            n102 = case shown="\"Mako G-158B (12750)\"" w266 {
              tunnel: w264 -> [w279 w287 w293 w299 w311 _]
              tunnel: w263 -> [w276 w286 w295 w298 w310 w322]
              tunnel: [w275 w285 w294 w297 w309 w321] -> w262
              frame "acA640-120gm" {
                n103 = Bundle By Name(cluster=T9 {"Minimum"=0.0, "Maximum"=0.0, "Increment"=0.0} ("Limites d'entrée des données"), "Minimum"=100.0, "Maximum"=1023.0, "Increment"=1.0) -> (w277:T9)
                n104 = property class="NumNb (strict)"(reference=w279, error in=w276, "Data Range"=w277) -> (error out=w275:errorcluster)  [unwired: 1 out]
              }
              frame "acA640-121gm" {
                n105 = Bundle By Name(cluster=T9 {"Minimum"=0.0, "Maximum"=0.0, "Increment"=0.0} ("Limites d'entrée des données"), "Minimum"=0.0, "Maximum"=1023.0, "Increment"=1.0) -> (w283:T9)
                n106 = property class="NumNb (strict)"(reference=w287, error in=w286, "Data Range"=w283) -> (error out=w285:errorcluster)  [unwired: 1 out]
              }
              frame "acA645-100gm" {
                n107 = Bundle By Name(cluster=T9 {"Minimum"=0.0, "Maximum"=0.0, "Increment"=0.0} ("Limites d'entrée des données"), "Minimum"=100.0, "Maximum"=1023.0, "Increment"=1.0) -> (w292:T9)
                n108 = property class="NumNb (strict)"(reference=w293, error in=w295, "Data Range"=w292) -> (error out=w294:errorcluster)  [unwired: 1 out]
              }
              frame "acA1600-60gm" {
                n109 = disable-structure shown="Activé" {
                  disable-tunnel: w299 -> [w307 _]
                  disable-tunnel: w298 -> [w306 w308]
                  disable-tunnel: [w305 w308] -> w297
                  disable-tunnel: T9 {"Minimum"=0.0, "Maximum"=0.0, "Increment"=0.0} ("Limites d'entrée des données") -> [w304 _]
                  frame Enabled {
                    n110 = Bundle By Name(cluster=w304, "Minimum"=0.0, "Maximum"=95.0, "Increment"=1.0) -> (w303:T9)
                    n111 = property class="NumNb (strict)"(reference=w307, error in=w306, "Data Range"=w303) -> (error out=w305:errorcluster)  [unwired: 1 out]
                  }
                  frame Disabled {
                  }
                }
              }
              frame "Mako G-158B (12750)" {
                n112 = disable-structure shown="Activé" {
                  disable-tunnel: w311 -> [w319 _]
                  disable-tunnel: w310 -> [w318 w320]
                  disable-tunnel: [w317 w320] -> w309
                  frame Enabled {
                    n113 = Bundle By Name(cluster=T9 {"Minimum"=0.0, "Maximum"=0.0, "Increment"=0.0} ("Limites d'entrée des données"), "Minimum"=0.0, "Maximum"=40.0, "Increment"=1.0) -> (w315:T9)
                    n114 = property class="NumNb (strict)"(reference=w319, error in=w318, "Data Range"=w315) -> (error out=w317:errorcluster)  [unwired: 1 out]
                  }
                  frame Disabled {
                  }
                }
              }
              frame Default {
                n115 = call <vilib>:"Simple Error Handler.vi"("error in (no error)"=w322) -> ("error out"=w321:errorcluster)  [unwired: 4 in, 4 out]
              }
            }
          }
        }
        n116 = call-dynamic "Error Handler.vi"("Worker"=w46, "error_in"=w48) -> ("error out"=w51:errorcluster, "Stop Loop"=w43:bool, "Worker out"=w50:refnum<class "UI Cam Basler.lvclass">)  [unwired: 7 in]
      }
      n117 = call-dynamic "Setup EHL.vi"("Worker"=w34) -> ("Worker out"=w35:refnum<class "UI Cam Basler.lvclass">)  [unwired: 14 in]
      n118 = while "Event Handling Loop" {
        shift-right: [w331] -> w38
        shift-left: w39 -> [w330]
        tunnel: [w326] -> w36
        tunnel: errorcluster {"status"=FALSE, "code"=0, "source"=""} ("error constant") -> [w328]
        shift-right: [w324] -> _
        shift-left: w35 -> [w329]
        stop <- w323 stop-if-true
        # "Event Handling Loop"
        n119 = event shown="[7] \"Image\": Souris relâchée" {
          selector: w330 -> [_ _ _ _ _ _ _ _ _ _ _ _ _]
          dyn-events: [_ _ _ _ _ _ _ _ _ _ _ _ _] -> w331
          timeout: _ -> [_ _ _ _ _ _ _ _ _ _ _ _ _]
          tunnel: [w335 w342 w355 w360 w366 w372 w378 w383 w388 w394 w398 w404 w410] -> w327
          tunnel: w328 -> [w336 w341 w356 w361 w367 w373 w379 w384 w389 w395 w399 w405 w411]
          tunnel: w329 -> [w334 w340 w354 w359 w365 w371 w377 w382 w387 w393 w397 w403 w409]
          tunnel: [w333 w339 w353 w358 w364 w370 w376 w381 w386 w392 w396 w402 w408] -> w325
          event User Event {
            # "This case and its contents must always be included in every EHL that you use, so that the framework can automatically stop the EHL."
            # "EHL Stop Event. This EHL exits from this case."
            n120 = event-data() -> ("Stop Event Data"=w332:variant)  [unwired: 1 in]
            n121 = call <vilib>:"EHL Stop - EHL Case.vi"("error in"=w336, "Stop Event Data"=w332, "Worker"=w334) -> ("error out"=w335:errorcluster, "Worker out"=w333:refnum<class "UI Cam Basler.lvclass">)  [unwired: 7 in]
          }
          event Panel Close? {
            # "Calls the Start Exiting case of this Worker. This will start the exiting sequence of this Worker."
            n122 = event-data() -> ()  [unwired: 1 in, 1 out]
            n123 = call <vilib>:"Read Queue.vi"("Worker"=w340) -> ("Message Queue out"=w337:refnum<class "Message Queue.lvclass">, "dup Worker out"=w338:refnum<class "UI Cam Basler.lvclass">)  [unwired: 9 in]
            n124 = disable-structure shown="Activé" {
              disable-tunnel: [w348 w350] -> w342
              disable-tunnel: w341 -> [w347 w350]
              disable-tunnel: [w346 w349] -> w339
              disable-tunnel: w338 -> [w345 w349]
              disable-tunnel: w337 -> [w344 _]
              frame Disabled {
                n125 = call-dynamic "Worker Start Exiting.vi"("error_in"=w347, "Message Queue"=w344, "Worker"=w345) -> ("error out"=w348:errorcluster, "dup Worker out"=w346:refnum<class "UI Cam Basler.lvclass">)  [unwired: 7 in]
              }
              frame Enabled {
              }
            }
            n126 = event-data("Discard?"=TRUE) -> ()  [unwired: 1 in, 1 out]
          }
          event Value Change {
            # "Camera name update"
            n127 = event-data() -> ("NewVal"=w352:T3)  [unwired: 1 in]
            n128 = call "c_update camera name.vi"() -> ("Case Label"=w351:T13)  [unwired: 1 in]
            n129 = call-poly <vilib>:"Enqueue Standard Message.vi"("Worker"=w354, "error in"=w356, "Data"=w352, "Case Label"=w351) -> ("error out"=w355:errorcluster, "dup Worker out"=w353:refnum<class "UI Cam Basler.lvclass">)  [unwired: 6 in]
          }
          event "Start": Value Change {
            # "Start Acquisition"
            n130 = event-data() -> ()  [unwired: 1 in, 1 out]
            n131 = call "c_Start.vi"() -> ("Case Label"=w357:T13)  [unwired: 1 in]
            n132 = call-poly <vilib>:"Enqueue Standard Message.vi"("Worker"=w359, "error in"=w361, "Case Label"=w357) -> ("error out"=w360:errorcluster, "dup Worker out"=w358:refnum<class "UI Cam Basler.lvclass">)  [unwired: 7 in]
          }
          event "Gain": Value Change {
            n133 = event-data() -> ("NewVal"=w363:dbl)  [unwired: 1 in]
            n134 = call "c_Update Gain.vi"() -> ("Case Label"=w362:T13)  [unwired: 1 in]
            n135 = call-poly <vilib>:"Enqueue Standard Message.vi"("Worker"=w365, "error in"=w367, "Data"=w363, "Case Label"=w362) -> ("error out"=w366:errorcluster, "dup Worker out"=w364:refnum<class "UI Cam Basler.lvclass">)  [unwired: 6 in]
          }
          event "Shutter(us)": Value Change {
            n136 = event-data() -> ("NewVal"=w369:dbl)  [unwired: 1 in]
            n137 = call "c_Update shutter.vi"() -> ("Case Label"=w368:T13)  [unwired: 1 in]
            n138 = call-poly <vilib>:"Enqueue Standard Message.vi"("Worker"=w371, "error in"=w373, "Data"=w369, "Case Label"=w368) -> ("error out"=w372:errorcluster, "dup Worker out"=w370:refnum<class "UI Cam Basler.lvclass">)  [unwired: 6 in]
          }
          event "ROI": Value Change {
            n139 = event-data() -> ("NewVal"=w375:bool)  [unwired: 1 in]
            n140 = call "c_Update ROI.vi"() -> ("Case Label"=w374:T13)  [unwired: 1 in]
            n141 = call-poly <vilib>:"Enqueue Standard Message.vi"("Worker"=w377, "error in"=w379, "Data"=w375, "Case Label"=w374) -> ("error out"=w378:errorcluster, "dup Worker out"=w376:refnum<class "UI Cam Basler.lvclass">)  [unwired: 6 in]
          }
          event "Image": Mouse Up {
            # "sauvegarde le ROI"
            n142 = event-data() -> ()  [unwired: 1 in, 1 out]
            n143 = call "c_Save pos ROI.vi"() -> ("Case Label"=w380:T13)  [unwired: 1 in]
            n144 = call-poly <vilib>:"Enqueue Standard Message.vi"("Worker"=w382, "error in"=w384, "Case Label"=w380) -> ("error out"=w383:errorcluster, "dup Worker out"=w381:refnum<class "UI Cam Basler.lvclass">)  [unwired: 7 in]
          }
          event Mouse Down {
            n145 = event-data() -> ()  [unwired: 1 in, 1 out]
            n146 = call "c_Set Splitter Bar.vi"() -> ("Case Label"=w385:T13)  [unwired: 1 in]
            n147 = call-poly <vilib>:"Enqueue Standard Message.vi"("Worker"=w387, "error in"=w389, "Case Label"=w385) -> ("error out"=w388:errorcluster, "dup Worker out"=w386:refnum<class "UI Cam Basler.lvclass">)  [unwired: 7 in]
          }
          event "Palette": Value Change {
            n148 = event-data() -> ("NewVal"=w391:u32)  [unwired: 1 in]
            n149 = call "c_Update image Palette.vi"() -> ("Case Label"=w390:T13)  [unwired: 1 in]
            n150 = call-poly <vilib>:"Enqueue Standard Message.vi"("Worker"=w393, "error in"=w395, "Data"=w391, "Case Label"=w390) -> ("error out"=w394:errorcluster, "dup Worker out"=w392:refnum<class "UI Cam Basler.lvclass">)  [unwired: 6 in]
          }
          event "Save Config": Value Change {
            # "Sauvegarde de la config d'acquisition"
            n151 = event-data() -> ()  [unwired: 1 in, 1 out]
            n152 = call "c_Save Configuration.vi"() -> ("Case Label"=w400:T13)  [unwired: 1 in]
            n153 = call-poly <vilib>:"Enqueue Standard Message.vi"("Worker"=w397, "error in"=w399, "Case Label"=w400) -> ("error out"=w398:errorcluster, "dup Worker out"=w396:refnum<class "UI Cam Basler.lvclass">)  [unwired: 7 in]
          }
          event "Stop": Value Change {
            # "Stop Acquisition"
            n154 = event-data() -> ()  [unwired: 1 in, 1 out]
            n155 = call "c_Stop.vi"() -> ("Case Label"=w401:T13)  [unwired: 1 in]
            n156 = call-poly <vilib>:"Enqueue Standard Message.vi"("Worker"=w403, "error in"=w405, "Case Label"=w401) -> ("error out"=w404:errorcluster, "dup Worker out"=w402:refnum<class "UI Cam Basler.lvclass">)  [unwired: 7 in]
          }
          event "toolbar?": Value Change {
            # "Update Toolbar"
            n157 = event-data() -> ("NewVal"=w406:bool)  [unwired: 1 in]
            n158 = call "c_Update Toolbar.vi"() -> ("Case Label"=w407:T13)  [unwired: 1 in]
            n159 = call-poly <vilib>:"Enqueue Standard Message.vi"("Worker"=w409, "error in"=w411, "Data"=w406, "Case Label"=w407) -> ("error out"=w410:errorcluster, "dup Worker out"=w408:refnum<class "UI Cam Basler.lvclass">)  [unwired: 6 in]
          }
        }
        n160 = call-dynamic "Error Handler.vi"("Worker"=w325, "error_in"=w327) -> ("error out"=w326:errorcluster, "Stop Loop"=w323:bool, "Worker out"=w324:refnum<class "UI Cam Basler.lvclass">)  [unwired: 7 in]
      }
    }
    frame Error {
      n161 = call-dynamic "Error Handler.vi"("Worker"=w413, "error_in"=w416) -> ("error out"=w414:errorcluster, "Worker out"=w412:refnum<class "UI Cam Basler.lvclass">)  [unwired: 7 in, 1 out]
    }
  }
  n162 = while {
    tunnel: w12 -> [w421]
    stop <- w420 stop-if-true
    n163 = Wait on Notification(notifier=w421) -> (notification=w419:T4, error out=w420:errorcluster)  [unwired: 3 in, 2 out]
    n164 = Unbundle By Name(w419) -> ("Image Out"=→"Image":T1, "FPS"=→"FPS":dbl)
  }
  n165 = call-dynamic "Main.vi"("error in"=w16, "Acq Cam Basler in"=w22) -> ("error out"=w19:errorcluster)  [unwired: 8 in, 1 out]
  n166 = Merge Errors(w19) -> (w18:errorcluster)
  n167 = Unregister For Events(event registration refnum=w29, error in=w30) -> (error out=w31:errorcluster)
  n168 = Merge Errors(w31, w24, w18) -> (w28:errorcluster)
  n169 = call-dynamic "Exited Notify and Cleanup.vi"("error_in"=w28, "Worker"=w27) -> ("error out"=→"error out":errorcluster, "dup Worker out"=→"UI Cam Basler out":refnum<class "UI Cam Basler.lvclass">)  [unwired: 8 in]
